vi "Get All Library Classes.vi"(8 "error in":errorcluster, 11 "library ref":refnum<vi>) -> (0 "error out":errorcluster, 3 "class refs":refnum<vi>[](array[refnum]))   [LabVIEW 2027, in "Build Automation.lvlib"]
uses:
  Build Automation.lvlib
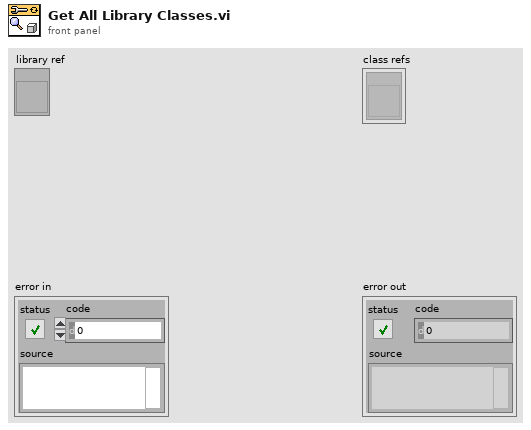
[diagram p1: front panel]
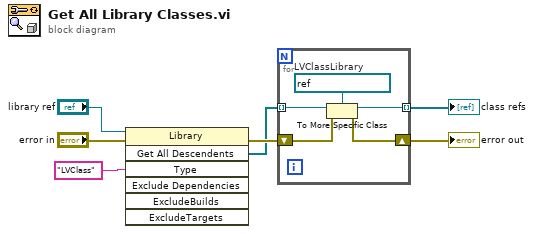
[diagram p0: block diagram]
diagram:
  n1 = invoke class="Library" method="Get All Descendents"(reference="library ref", error in="error in", "Type"="LVClass" ("y")) -> (error out=w6:errorcluster, "All Descendents"=w5:refnum<vi>[])  [unwired: 4 in, 5 out]
  n2 = for {
    shift-right: [w9] -> w3
    shift-left: w6 -> [w10]
    tunnel: w5 -> [w12] mode=indexing
    tunnel: [w8] -> w2 mode=indexing
    w11 = refnum<vi> refnum  # LVClassLibrary
    n3 = To More Specific Class(target class=w11, reference=w12, error in=w10) -> (specific class reference=w8:refnum<vi>, error out=w9:errorcluster)
  }
  "error out" <- w3
  "class refs" <- w2
